vi "test.run.all.vi"() -> ()   [LabVIEW 2020]
panel:
  out "Passed":bool
  out "# of Results":i32
  out "Results":bool[](array[boolean])
  out "Get All Control Values Variant":T1(array[cluster])
  out "Array":path[](array[path])
  out "error out":errorcluster
  in  "error in":errorcluster
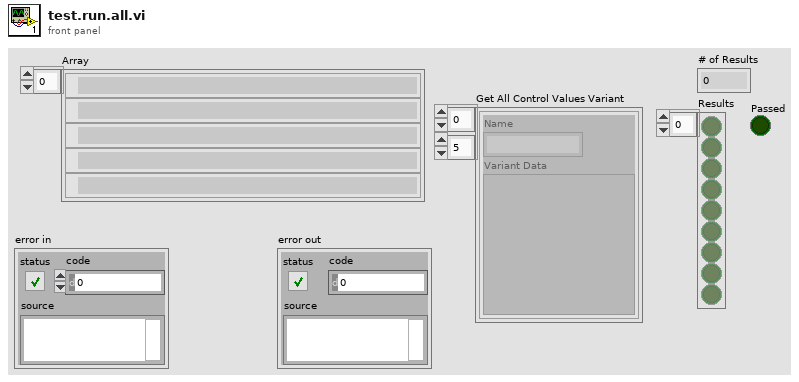
[diagram p1: front panel]
types:
  T1 = cluster{"Name":string, "Variant Data":variant}[][]
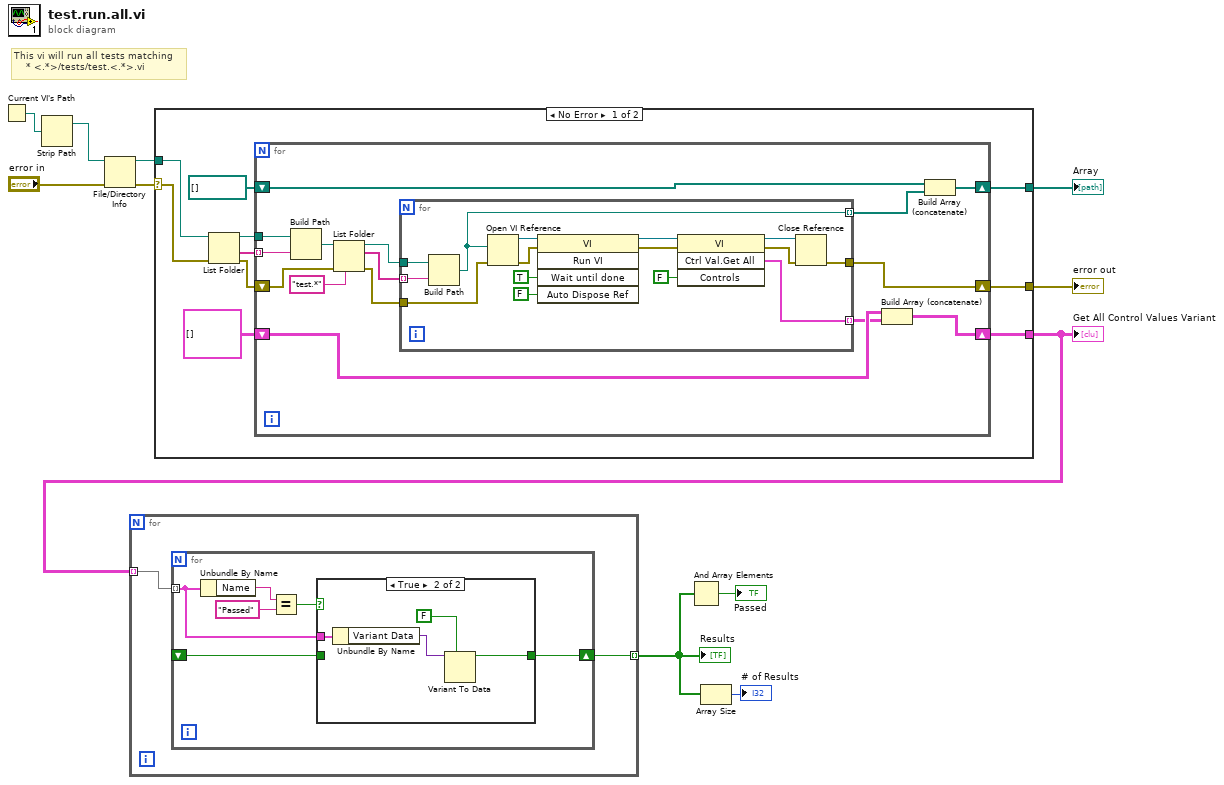
[diagram p0: block diagram]
diagram:
  # "This vi will run all tests matching\n    * <.*>/tests/test.<.*>.vi"
  n1 = Current VI's Path() -> (path=w2:path)
  n2 = Strip Path(path=w2) -> (stripped path=w1:path)  [unwired: 1 out]
  n3 = File/Directory Info(path=w1, error in="error in") -> (path out=w3:path, error out=w10:errorcluster)  [unwired: 5 out]
  n4 = case shown="No Error" w10 {
    selector: w10 -> [w21 w52]
    tunnel: [w19 _] -> w9
    tunnel: [w17 w52] -> w8
    tunnel: [w16 _] -> w7
    tunnel: w3 -> [w15 _]
    frame No Error {
      n5 = List Folder(path=w15, error in=w21) -> (path out=w20:path, folder names=w14:string[], error out=w18:errorcluster)  [unwired: 2 in, 1 out]
      n6 = for {
        tunnel: w20 -> [w36]
        shift-right: [w22] -> w17
        shift-left: w18 -> [w33]
        tunnel: w14 -> [w35] mode=indexing
        shift-right: [w31] -> w19
        shift-left: path[] [] -> [w32]
        shift-right: [w25] -> w16
        shift-left: T1 [] ("Get All Control Values Variant 2") -> [w24]
        n7 = Build Path(base path=w36, name or relative path=w35) -> (appended path=w34:path)
        n8 = List Folder(path=w34, pattern="test.*", error in=w33) -> (path out=w29:path, filenames=w28:string[], error out=w26:errorcluster)  [unwired: 1 in, 1 out]
        n9 = for {
          tunnel: w29 -> [w51]
          tunnel: w28 -> [w50] mode=indexing
          tunnel: [w39] -> w27 mode=indexing
          tunnel: w26 -> [w40]
          tunnel: [w38] -> w23 mode=indexing
          tunnel: [w37] -> w22
          n10 = Build Path(base path=w51, name or relative path=w50) -> (appended path=w39:path)
          n11 = Open VI Reference(vi path=w39, error in (no error)=w40) -> (vi reference=w44:refnum<vi>, error out=w45:errorcluster)  [unwired: 4 in]
          n12 = invoke class="VI" method="Run VI"(reference=w44, error in=w45, "Wait until done"=TRUE ("Wait Until Done"), "Auto Dispose Ref"=FALSE ("Auto Dispose Reference")) -> (reference out=w46:refnum<vi>, error out=w48:errorcluster)  [unwired: 1 in, 3 out]
          n13 = invoke class="VI" method="Ctrl Val.Get All"(reference=w46, error in=w48, "Controls"=FALSE) -> (reference out=w47:refnum<vi>, error out=w49:errorcluster, "Get All Control Values Variant"=w38:cluster{"Name":string, "Variant Data":variant}[])  [unwired: 1 in, 1 out]
          n14 = Close Reference(reference=w47, error in (no error)=w49) -> (error out=w37:errorcluster)
        }
        n15 = Build Array (concatenate)(w24, w23) -> (w25:T1)
        n16 = Build Array (concatenate)(w32, w27) -> (w31:path[])
      }
    }
    frame Error {
    }
  }
  "error out" <- w8
  "Array" <- w9
  "Get All Control Values Variant" <- w7
  n17 = for {
    tunnel: w7 -> [w54] mode=indexing
    tunnel: [w53] -> w5 mode=indexing
    n18 = for {
      tunnel: w54 -> [w57] mode=indexing
      shift-right: [w56] -> w53
      shift-left: _ -> [w55]
      n19 = Unbundle By Name(w57) -> ("Name"=w60:string)
      n20 = Equal?(x=w60, y="Passed") -> (x = y?=w58:bool)
      n21 = case shown="True" w58 {
        tunnel: w57 -> [_ w65]
        tunnel: [w61 w62] -> w56
        tunnel: w55 -> [w61 _]
        frame False {
        }
        frame True {
          n22 = Unbundle By Name(w65) -> ("Variant Data"=w64:variant)
          n23 = Variant To Data(type=FALSE, Variant=w64) -> (data=w62:bool)  [unwired: 1 in, 1 out]
        }
      }
    }
  }
  "Results" <- w5
  n24 = And Array Elements(Boolean array=w5) -> (logical AND=→"Passed":bool)
  n25 = Array Size(array=w5) -> (size(s)=→"# of Results":i32)
